vi "PH_SHS_Analysis_Calibrator.ProcCases.vi"(0 "i ref in":refnum<vi>, 1 "selector":string, 2 "data":T1, 3 "call cluster":T2={"Object"="", "Selector"="", "CallType"=enum."synchronous", "Async Object"="", "Async Selector"="", "Data Descriptor"="", "Data"=[], "Error #"=0, "Expire"=0}, 5 "error in":errorcluster) -> (14 "i ref out":refnum<vi>, 17 "answer cluster":T2={"Object"="", "Selector"="", "CallType"=enum."synchronous", "Async Object"="", "Async Selector"="", "Data Descriptor"="", "Data"=[], "Error #"=0, "Expire"=0}, 19 "error out":errorcluster)   [LabVIEW 2014, in "PH_SHS_Analysis_Calibrator.lvlib"]
doc: "This method is called by a process from within the default case in the event loop. The methods of a class that are linked to events will be called from THIS method. Add your code here."
uses:
  PH_SHS_Analysis_Calibrator.lvlib
  CS_Core/CSSystem/CoreDefs/CoreDefs.call_type.ctl
  CS_Core/BaseProcess/BaseProcess.descriptor string definition.ctl
  CS_Core/CSSystem/CoreDefs/CoreDefs.rawDataType.ctl
  CS_Core/CSSystem/CoreLib/CoreLib.string 2 byte array.vi
  CS_Core/CSSystem/CoreLib/CoreLib.byte array 2 string.vi
  CS_Core/BaseProcess/BaseProcess.lvlib
  CS_Core/CSSystem/CoreLib/CoreLib.lvlib
  CS_Core/BaseSM/BaseSM.lvlib
  PH_Basics/PH_Img_BaseClass/PH_Img_BaseClass.lvlib
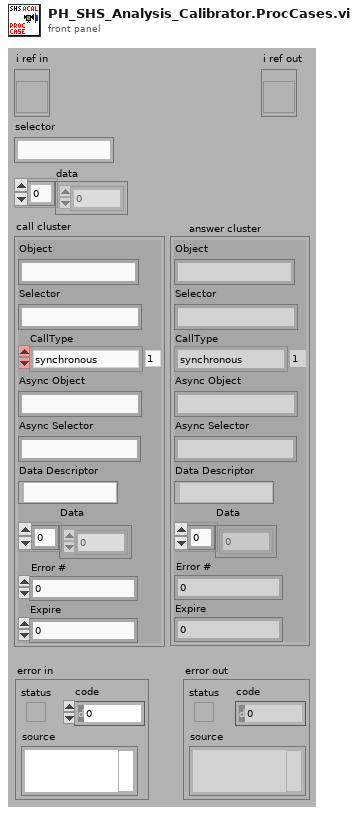
[diagram p1: front panel]
types:
  T1 = typedef "CoreDefs.rawDataType.ctl" = i8[]
  T2 = typedef "CoreDefs.call_type.ctl" = cluster{"Object":string, "Selector":string, "CallType":enum16{"simple", "synchronous", "asynchronous"}, "Async Object":string, "Async Selector":string, "Data Descriptor":T3, "Data":T1, "Error #":i32, "Expire":u32}
  T3 = typedef "BaseProcess.lvlib/BaseProcess.descriptor string definition.ctl" = string
  T4 = typedef "PH_SHS_Analysis_Calibrator.lvlib/PH_SHS_Analysis_Calibrator.i attribute.ctl" = cluster{"GUI Refs":cluster{"Available Cams":refnum<vi>, "OK":refnum<vi>, "Skip":refnum<vi>, "Repeat":refnum<vi>, "Cancel":refnum<vi>, "Dialog":refnum<vi>, "Enough Images?":refnum<vi>}, "Cam instances":string[], "Status":cluster{"#":i32, "Data calculated":bool, "Wanted #":i32}, "IMAQ Image Array":T5[], "Pixel Size [µm]":dbl, "MLA Pitch [µm]":dbl, "Method":enum16{"automatic", "manual"}, "Enough Images?":bool, "SHS Reference Result":T6, "Calculation Error":errorcluster}
  T5 = typedef "IMAQ Image.ctl" = refnum<image>
  T6 = typedef "SHS_Common.lvlib/SHSReference.ctl" = cluster{"Reference":T7[][], "Lens Array Pitch [px]":dbl}
  T7 = typedef "SHS_Common.lvlib/ReferencePoint.ctl" = cluster{"Rect":T8, "Point":T9}
  T8 = typedef "SHS_Common.lvlib/Rectangle.ctl" = cluster{"Left":i32, "Top":i32, "Right":i32, "Bottom":i32}
  T9 = typedef "SHS_Common.lvlib/Point.ctl" = cluster{"x":dbl, "y":dbl, "valid?":bool, "weight":dbl}
  T10 = typedef "PH_Img_BaseClass.lvlib/PH_Img_BaseClass.i attribute.ctl" = cluster{"GUI Refs":T11, "Timeout Image [ms]":i32, "Default Periodic Period [ms]":i32, "Camera":cluster{"Instancename":string, "Notifier":refnum<notifier>}, "Palette":T12, "Cam Settings":cluster{"Cam ID":string, "Gain":dbl, "Brightness":dbl, "Shutter":dbl, "Cam Info Failure":bool, "Mode":i32}}
  T11 = typedef "PH_Img_BaseClass.lvlib/PH_Img_BaseClass.GUI Refs.ctl" = cluster{"Timeout":refnum<vi>, "Image":refnum<vi>, "Palette":refnum<vi>, "Timeout Set":refnum<vi>}
  T12 = typedef "PH_Img_BaseClass.lvlib/PH_Img_BaseClass.Palette.ctl" = i32
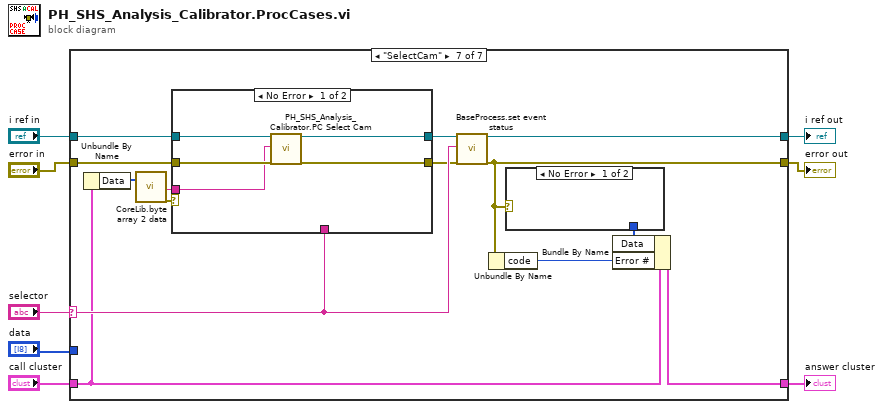
[diagram p0: block diagram]
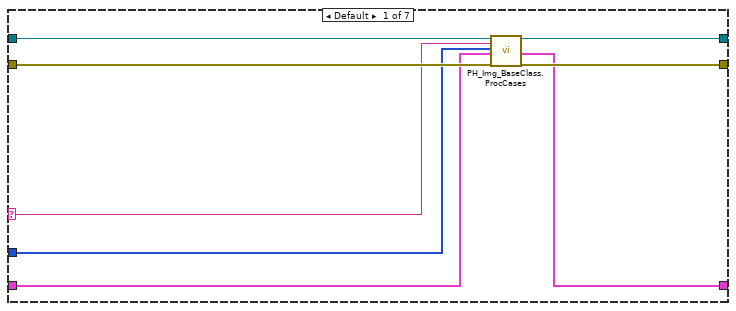
[diagram p2: hidden frame]
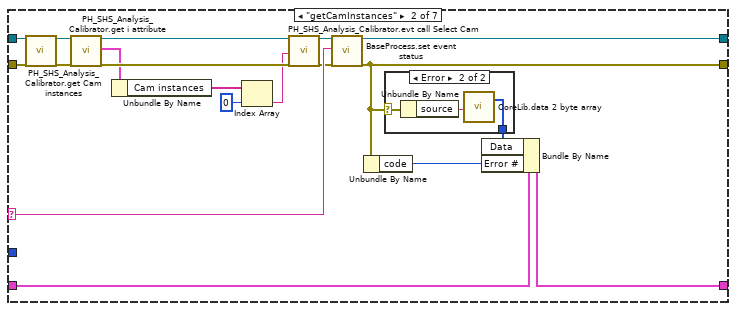
[diagram p3: hidden frame]
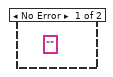
[diagram p4: hidden frame]
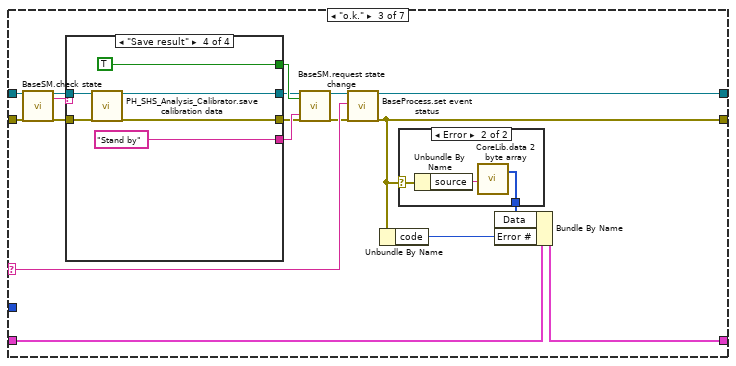
[diagram p5: hidden frame]
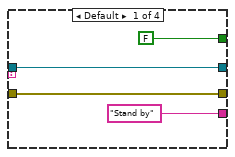
[diagram p6: hidden frame]
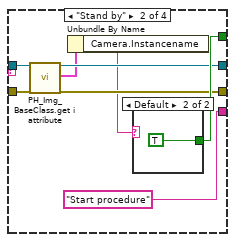
[diagram p7: hidden frame]
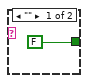
[diagram p8: hidden frame]
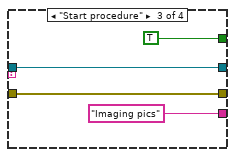
[diagram p9: hidden frame]
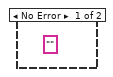
[diagram p10: hidden frame]
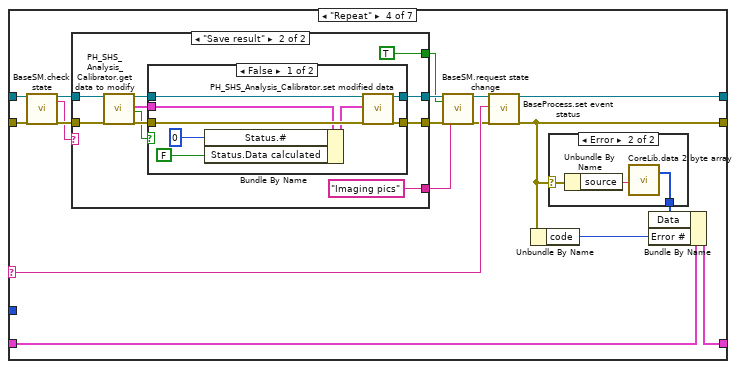
[diagram p11: hidden frame]
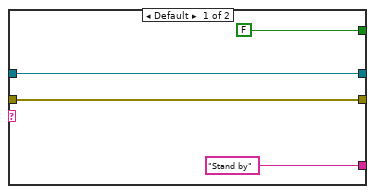
[diagram p12: hidden frame]
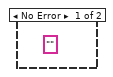
[diagram p14: hidden frame]
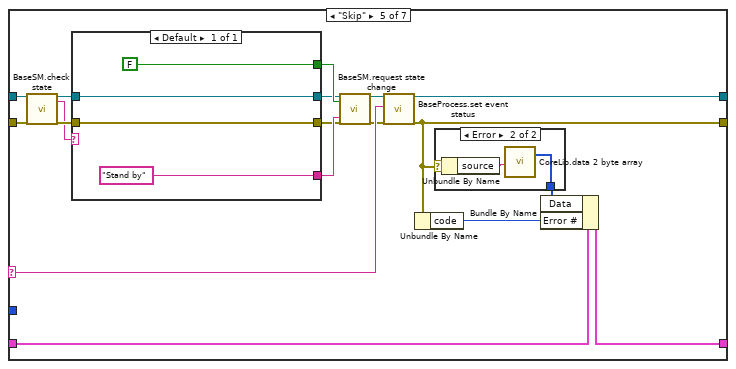
[diagram p15: hidden frame]
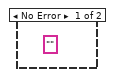
[diagram p16: hidden frame]
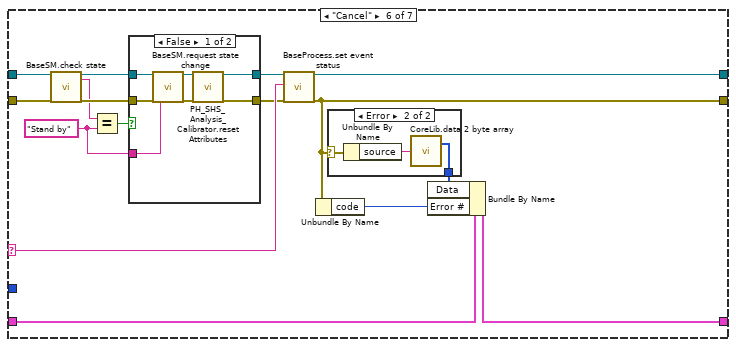
[diagram p17: hidden frame]
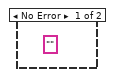
[diagram p19: hidden frame]
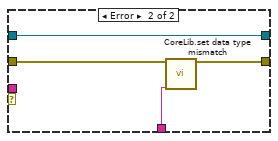
[diagram p20: hidden frame]
diagram:
  n1 = case shown="\"SelectCam\"" "selector" {
    selector: "selector" -> [w10 w31 w52 w97 w142 w165 w191]
    tunnel: "data" -> [w11 _ _ _ _ _ _]
    tunnel: "i ref in" -> [w9 w29 w50 w93 w138 w159 w189]
    tunnel: [w16 w30 w51 w96 w141 w164 w192] -> w4
    tunnel: "call cluster" -> [w12 w34 w55 w100 w145 w168 w190]
    tunnel: [w13 w33 w54 w99 w144 w167 w194] -> w7
    tunnel: "error in" -> [w15 w28 w49 w92 w137 w161 w187]
    tunnel: [w14 w32 w53 w98 w143 w166 w193] -> w3
    frame Default {
      n2 = call "PH_Img_BaseClass.ProcCases.vi"("i ref in"=w9, "selector"=w10, "Data"=w11, "call cluster"=w12, "error in (no error)"=w15) -> ("i ref out"=w16:refnum<vi>, "answer cluster"=w13:T2, "error out"=w14:errorcluster)  [unwired: 12 in]
    }
    frame "getCamInstances" {
      n3 = call "PH_SHS_Analysis_Calibrator.get Cam instances.vi"("i ref in"=w29, "error in"=w28) -> ("i ref out"=w27:refnum<vi>, "error out"=w24:errorcluster)  [unwired: 16 in]
      n4 = call "PH_SHS_Analysis_Calibrator.get i attribute.vi"("i ref in"=w27, "error in (no error)"=w24) -> ("i ref out"=w18:refnum<vi>, "i attribute"=w22:T4, "error out"=w25:errorcluster)  [unwired: 15 in]
      n5 = Unbundle By Name(w22) -> ("Cam instances"=w21:string[])
      n6 = Index Array(array=w21, index=0) -> (element=w19:string)
      n7 = call "PH_SHS_Analysis_Calibrator.evt call Select Cam.vi"("i ref in"=w18, "Cam"=w19, "error in"=w25) -> ("i ref out"=w26:refnum<vi>, "error out"=w23:errorcluster)  [unwired: 15 in]
      n8 = call "BaseProcess.set event status.vi"("i ref in"=w26, "EventStatus"=w31, "error in (no error)"=w23) -> ("i ref out"=w30:refnum<vi>, "error out"=w32:errorcluster)  [unwired: 14 in, 1 out]
      n9 = Unbundle By Name(w32) -> ("code"=w35:i32)
      n10 = case shown="Error" w32 {
        selector: w32 -> [_ w38]
        tunnel: [_ w36] -> w17
        frame No Error {
          (unwired) "" ("source")
        }
        frame Error {
          n11 = Unbundle By Name(w38) -> ("source"=w37:string)
          n12 = call-poly "CoreLib.data 2 byte array.vi"("string"=w37) -> ("byteArray out"=w36:T1)  [unwired: 18 in]
        }
      }
      n13 = Bundle By Name(cluster=w34, "Data"=w17, "Error #"=w35) -> (w33:T2)
    }
    frame "o.k." {
      n14 = call "BaseSM.check state.vi"("i ref in"=w50, "error in (no error)"=w49) -> ("i ref out"=w43:refnum<vi>, "actualState"=w44:string, "error out"=w41:errorcluster)  [unwired: 12 in, 3 out]
      n15 = case shown="\"Save result\"" w44 {
        tunnel: ["Stand by" ("requested state") "Start procedure" ("requested state") "Imaging pics" ("requested state") "Stand by" ("requested state")] -> w46
        tunnel: [FALSE ("change") w67 TRUE ("change") TRUE ("change")] -> w45
        tunnel: w43 -> [w58 w66 w72 w78]
        tunnel: [w58 w65 w72 w77] -> w42
        tunnel: w41 -> [w57 w64 w71 w76]
        tunnel: [w57 w63 w71 w75] -> w40
        frame Default {
        }
        frame "Stand by" {
          n16 = call "PH_Img_BaseClass.get i attribute.vi"("i ref in"=w66, "error in (no error)"=w64) -> ("i ref out"=w65:refnum<vi>, "i attribute"=w62:T10, "error out"=w63:errorcluster)  [unwired: 15 in]
          n17 = Unbundle By Name(w62) -> ("Camera.Instancename"=w61:string)
          n18 = case shown="Default" w61 {
            tunnel: [FALSE TRUE ("change")] -> w67
            frame "" {
            }
            frame Default {
            }
          }
        }
        frame "Start procedure" {
        }
        frame "Save result" {
          n19 = call "PH_SHS_Analysis_Calibrator.save calibration data.vi"("i ref in"=w78, "error in (no error)"=w76) -> ("i ref out"=w77:refnum<vi>, "error out"=w75:errorcluster)  [unwired: 16 in]
        }
      }
      n20 = call "BaseSM.request state change.vi"("i ref in"=w42, "change"=w45, "error in (no error)"=w40, "requested state"=w46) -> ("i ref out"=w48:refnum<vi>, "error out"=w47:errorcluster)  [unwired: 12 in, 2 out]
      n21 = call "BaseProcess.set event status.vi"("i ref in"=w48, "EventStatus"=w52, "error in (no error)"=w47) -> ("i ref out"=w51:refnum<vi>, "error out"=w53:errorcluster)  [unwired: 14 in, 1 out]
      n22 = Unbundle By Name(w53) -> ("code"=w56:i32)
      n23 = case shown="Error" w53 {
        selector: w53 -> [_ w83]
        tunnel: [_ w82] -> w39
        frame No Error {
          (unwired) "" ("source")
        }
        frame Error {
          n24 = Unbundle By Name(w83) -> ("source"=w81:string)
          n25 = call-poly "CoreLib.data 2 byte array.vi"("string"=w81) -> ("byteArray out"=w82:T1)  [unwired: 18 in]
        }
      }
      n26 = Bundle By Name(cluster=w55, "Data"=w39, "Error #"=w56) -> (w54:T2)
    }
    frame "Repeat" {
      n27 = call "BaseSM.check state.vi"("i ref in"=w93, "error in (no error)"=w92) -> ("i ref out"=w95:refnum<vi>, "actualState"=w91:string, "error out"=w94:errorcluster)  [unwired: 12 in, 3 out]
      n28 = case shown="\"Save result\"" w91 {
        tunnel: [w105 w106] -> w87
        tunnel: [w104 w108] -> w89
        tunnel: w95 -> [w105 w107]
        tunnel: w94 -> [w104 w109]
        tunnel: [FALSE TRUE] -> w86
        tunnel: ["Stand by" "Imaging pics"] -> w85
        frame Default {
        }
        frame "Save result" {
          n29 = call "PH_SHS_Analysis_Calibrator.get data to modify.vi"("i ref in"=w107, "error in (no error)"=w109) -> ("i ref out"=w113:refnum<vi>, "i attribute"=w111:T4, "timed out"=w110:bool, "error out"=w112:errorcluster)  [unwired: 14 in]
          n30 = case shown="False" w110 {
            tunnel: w113 -> [w123 w125]
            tunnel: w112 -> [w122 w124]
            tunnel: [w121 w125] -> w106
            tunnel: [w120 w124] -> w108
            tunnel: w111 -> [w119 _]
            frame False {
              n31 = Bundle By Name(cluster=w119, "Status.#"=0, "Status.Data calculated"=FALSE ("Energy Cali.Underground subtracted?")) -> (w118:T4)
              n32 = call "PH_SHS_Analysis_Calibrator.set modified data.vi"("i ref in"=w123, "i attribute"=w118, "error in (no error)"=w122) -> ("i ref out"=w121:refnum<vi>, "error out"=w120:errorcluster)  [unwired: 15 in]
            }
            frame True {
            }
          }
        }
      }
      n33 = call "BaseSM.request state change.vi"("i ref in"=w87, "change"=w86, "error in (no error)"=w89, "requested state"=w85) -> ("i ref out"=w88:refnum<vi>, "error out"=w90:errorcluster)  [unwired: 12 in, 2 out]
      n34 = call "BaseProcess.set event status.vi"("i ref in"=w88, "EventStatus"=w97, "error in (no error)"=w90) -> ("i ref out"=w96:refnum<vi>, "error out"=w98:errorcluster)  [unwired: 14 in, 1 out]
      n35 = Unbundle By Name(w98) -> ("code"=w101:i32)
      n36 = case shown="Error" w98 {
        selector: w98 -> [_ w128]
        tunnel: [_ w126] -> w84
        frame No Error {
          (unwired) "" ("source")
        }
        frame Error {
          n37 = Unbundle By Name(w128) -> ("source"=w127:string)
          n38 = call-poly "CoreLib.data 2 byte array.vi"("string"=w127) -> ("byteArray out"=w126:T1)  [unwired: 18 in]
        }
      }
      n39 = Bundle By Name(cluster=w100, "Data"=w84, "Error #"=w101) -> (w99:T2)
    }
    frame "Skip" {
      n40 = call "BaseSM.check state.vi"("i ref in"=w138, "error in (no error)"=w137) -> ("i ref out"=w140:refnum<vi>, "actualState"=w136:string, "error out"=w139:errorcluster)  [unwired: 12 in, 3 out]
      n41 = case shown="Default" w136 {
        tunnel: [w150] -> w132
        tunnel: [w149] -> w130
        tunnel: w140 -> [w150]
        tunnel: w139 -> [w149]
        tunnel: ["Stand by" ("requested state")] -> w135
        tunnel: [FALSE] -> w134
        frame Default {
        }
      }
      n42 = call "BaseSM.request state change.vi"("i ref in"=w132, "change"=w134, "error in (no error)"=w130, "requested state"=w135) -> ("i ref out"=w133:refnum<vi>, "error out"=w131:errorcluster)  [unwired: 12 in, 2 out]
      n43 = call "BaseProcess.set event status.vi"("i ref in"=w133, "EventStatus"=w142, "error in (no error)"=w131) -> ("i ref out"=w141:refnum<vi>, "error out"=w143:errorcluster)  [unwired: 14 in, 1 out]
      n44 = Unbundle By Name(w143) -> ("code"=w146:i32)
      n45 = case shown="Error" w143 {
        selector: w143 -> [_ w153]
        tunnel: [_ w151] -> w129
        frame No Error {
          (unwired) "" ("source")
        }
        frame Error {
          n46 = Unbundle By Name(w153) -> ("source"=w152:string)
          n47 = call-poly "CoreLib.data 2 byte array.vi"("string"=w152) -> ("byteArray out"=w151:T1)  [unwired: 18 in]
        }
      }
      n48 = Bundle By Name(cluster=w145, "Data"=w129, "Error #"=w146) -> (w144:T2)
    }
    frame "Cancel" {
      w155 = "Stand by" ("y")
      n49 = call "BaseSM.check state.vi"("i ref in"=w159, "error in (no error)"=w161) -> ("i ref out"=w158:refnum<vi>, "actualState"=w156:string, "error out"=w160:errorcluster)  [unwired: 12 in, 3 out]
      n50 = Equal?(x=w156, y=w155) -> (x = y?=w157:bool)
      n51 = case shown="False" w157 {
        tunnel: [w176 w178] -> w163
        tunnel: [w175 w177] -> w162
        tunnel: w160 -> [w174 w177]
        tunnel: w158 -> [w172 w178]
        tunnel: w155 -> [w170 _]
        frame False {
          n52 = call "BaseSM.request state change.vi"("i ref in"=w172, "error in (no error)"=w174, "requested state"=w170) -> ("i ref out"=w171:refnum<vi>, "error out"=w173:errorcluster)  [unwired: 13 in, 2 out]
          n53 = call "PH_SHS_Analysis_Calibrator.reset Attributes.vi"("i ref in"=w171, "error in (no error)"=w173) -> ("i ref out"=w176:refnum<vi>, "error out"=w175:errorcluster)  [unwired: 16 in]
        }
        frame True {
        }
      }
      n54 = call "BaseProcess.set event status.vi"("i ref in"=w163, "EventStatus"=w165, "error in (no error)"=w162) -> ("i ref out"=w164:refnum<vi>, "error out"=w166:errorcluster)  [unwired: 14 in, 1 out]
      n55 = Unbundle By Name(w166) -> ("code"=w169:i32)
      n56 = case shown="Error" w166 {
        selector: w166 -> [_ w181]
        tunnel: [_ w179] -> w154
        frame No Error {
          (unwired) "" ("source")
        }
        frame Error {
          n57 = Unbundle By Name(w181) -> ("source"=w180:string)
          n58 = call-poly "CoreLib.data 2 byte array.vi"("string"=w180) -> ("byteArray out"=w179:T1)  [unwired: 18 in]
        }
      }
      n59 = Bundle By Name(cluster=w168, "Data"=w154, "Error #"=w169) -> (w167:T2)
    }
    frame "SelectCam" {
      n60 = Unbundle By Name(w190) -> ("Data"=w185:T1)
      n61 = call-poly "CoreLib.byte array 2 data.vi"("byteArray"=w185) -> ("string"=w184:string, "error out"=w183:errorcluster)  [unwired: 16 in, 1 out]
      n62 = case shown="No Error" w183 {
        tunnel: w189 -> [w200 w202]
        tunnel: [w196 w202] -> w188
        tunnel: w187 -> [w199 w204]
        tunnel: [w197 w203] -> w186
        tunnel: w191 -> [_ w201]
        tunnel: w184 -> [w198 _]
        frame No Error {
          n63 = call "PH_SHS_Analysis_Calibrator.PC Select Cam.vi"("VI in"=w200, "Source"=w198, "error in (no error)"=w199) -> ("VI out"=w196:refnum<vi>, "error out"=w197:errorcluster)  [unwired: 15 in]
        }
        frame Error {
          n64 = call "CoreLib.set data type mismatch.vi"("error in (no error)"=w204, "error source"=w201) -> ("error out"=w203:errorcluster)  [unwired: 17 in]
        }
      }
      n65 = call "BaseProcess.set event status.vi"("i ref in"=w188, "EventStatus"=w191, "error in (no error)"=w186) -> ("i ref out"=w192:refnum<vi>, "error out"=w193:errorcluster)  [unwired: 14 in, 1 out]
      n66 = Unbundle By Name(w193) -> ("code"=w195:i32)
      n67 = case shown="No Error" w193 {
        selector: w193 -> [_ w207]
        tunnel: [_ w205] -> w182
        frame No Error {
        }
        frame Error {
          n68 = Unbundle By Name(w207) -> ("source"=w206:string)
          n69 = call-poly "CoreLib.data 2 byte array.vi"("string"=w206) -> ("byteArray out"=w205:T1)  [unwired: 18 in]
        }
      }
      n70 = Bundle By Name(cluster=w190, "Data"=w182, "Error #"=w195) -> (w194:T2)
    }
  }
  "answer cluster" <- w7
  "i ref out" <- w4
  "error out" <- w3
